vi "打印前面板R092B.vi"(0 "二维图片":picture) -> ()   [LabVIEW 2020]
uses:
  Sources/Global_Variable/Global.vi
panel:
  out "软件版本号 2":string
  out "软件版本号":string
  out "二维图片 2":picture
  # "P\n电动转向管柱\n带中间轴总成\n6HL S11-3404010"
  # "3404DB"
  # "H1.10"
  # "CHINA"
  # "P\n电动转向管柱\n带中间轴总成\n6HL S11-3404010"
  # "3404DB"
  # "H1.10"
  # "CHINA"
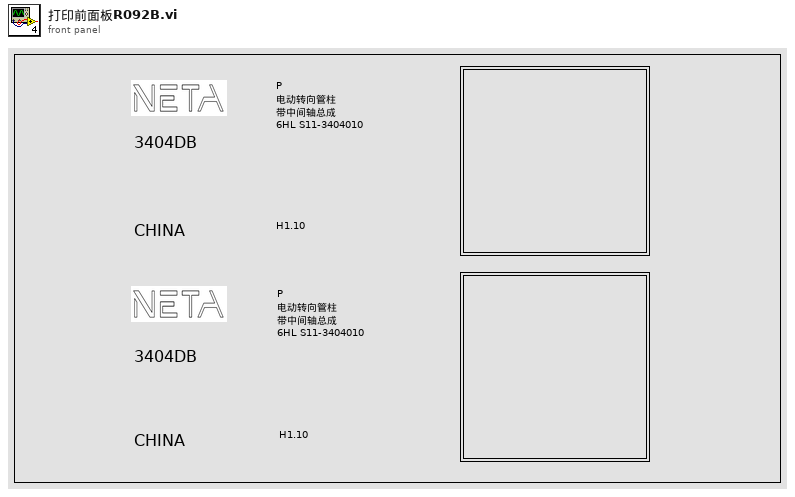
[diagram p1: front panel]
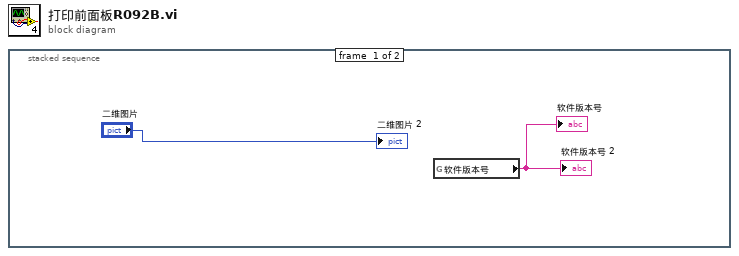
[diagram p0: block diagram]
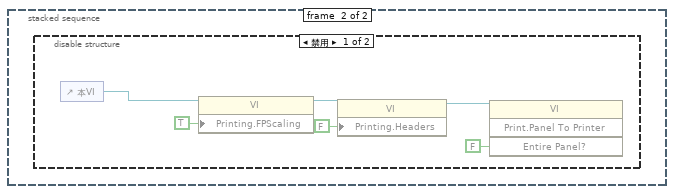
[diagram p2: hidden frame]
diagram:
  n1 = stacked-sequence {
    frame #0 {
      n2 = global read "Global.vi" "软件版本号"() -> (→"软件版本号" →"软件版本号 2":string)
      "二维图片 2" <- "二维图片"
    }
    frame #1 {
      n3 = disable-structure shown="禁用" {
        frame Disabled {
          n4 = control-ref of="本VI"() -> (w8:refnum<vi>)
          n5 = property class="VI"(reference=w8, "Printing.FPScaling"=TRUE ("打印:前面板缩放？")) -> (reference out=w6:refnum<vi>)  [unwired: 1 in, 1 out]
          n6 = property class="VI"(reference=w6, "Printing.Headers"=FALSE ("打印:页眉？")) -> (reference out=w4:refnum<vi>)  [unwired: 1 in, 1 out]
          n7 = invoke class="VI" method="Print.Panel To Printer"(reference=w4, "Entire Panel?"=FALSE ("整个前面板？")) -> ()  [unwired: 2 in, 4 out]
        }
        frame Enabled {
        }
      }
    }
  }
